vi "SYST_PREF_ITEM_PSRT.vi"(0 "VISA IN":refnum<visa-resource-name>, 5 "error in":errorcluster, 7 "Power":string(combo)="STARt") -> (14 "VISA Out":refnum<visa-resource-name>, 19 "error out":errorcluster)   [LabVIEW 2018, in "PNA-X.lvlib"]
doc: "SYSTem:PREFerences:ITEM:PSRTrace <char> \n(Read-Write) At the end of a power sweep, while waiting to trigger the next sweep, maintain source \npower at either the start power level or at the stop power level. \nTo send this command using the PNA front panel, open the GPIB Command Processor Console, then \ntype either of the following examples at the command prompt. Then type the Query Syntax and press \nenter to be sure the PNA took the command. \nThis setting remains until changed again using this command, or until the hard drive is changed or \nreformatted. \nParameters \n<char> Choose from: \nSTARt - Maintain source power at the start power level. \nSTOP - Maintain source power at the stop power level. \nExamples SYST:PREF:ITEM:PSRT STOP \nsystem:preferences:item:psrtrace start \nQuery Syntax SYSTem:PREFerences:ITEM:PSRTrace? \nReturn Type Character \nDefault STARt"
uses:
  PNA-X.lvlib
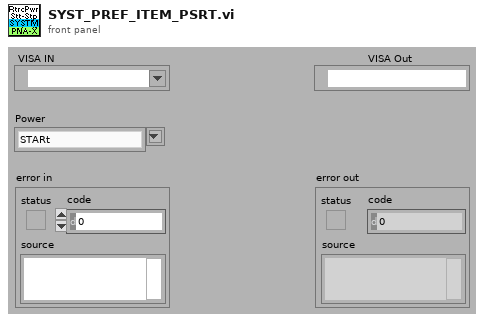
[diagram p1: front panel]
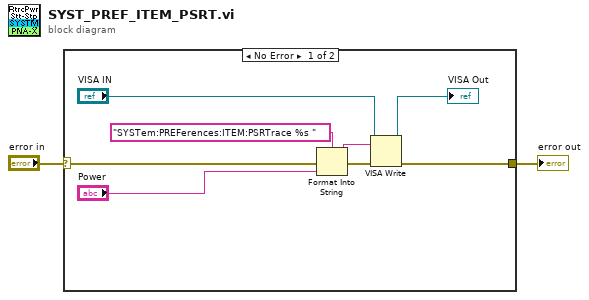
[diagram p0: block diagram]
diagram:
  n1 = case shown="No Error" "error in" {
    selector: "error in" -> [w10 w11]
    tunnel: [w5 w11] -> w1
    frame No Error {
      n2 = Format Into String(format string="SYSTem:PREFerences:ITEM:PSRTrace %s " ("Cmdline"), error in=w10, "Power") -> (resulting string=w8:string, error out=w9:errorcluster)  [unwired: 1 in]
      n3 = VISA Write(VISA resource name="VISA IN", write buffer=w8, error in (no error)=w9) -> (VISA resource name out=→"VISA Out":refnum<visa-resource-name>, error out=w5:errorcluster)  [unwired: 1 out]
    }
    frame Error {
    }
  }
  "error out" <- w1
